vi "Siglent SDG X Series Frequency Sweep.vi"() -> ()   [LabVIEW 2022 SP3]
doc: "This example shows how to configure and enable a frequency sweep."
uses:
  Siglent SDG X Series.lvlib
panel:
  in  "VISA resource name":refnum<visa-resource-name>
  in  "Stop Frequency  (1000.0 Hz)":dbl=1000.0 format="%#.6g"
  in  "Start Frequency (100.0 Hz)":dbl=100.0 format="%#.6g"
  in  "Sweep Time (1.00 s)":dbl=1.0 format="%#.6g"
  in  "Amplitude (1.0 Vpp)":dbl=1.0 format="%#.3f"
  in  "Waveform Function (0: Sine)":u16(ring) items=["Sine", "Square", "Ramp", "DC", "Pulse", "Arb"]
  in  "Channel (1:Channel 1)":i32(ring)=1 items=["Channel 1"=1, "Channel 2"=2]
  # "(c) 2017 SIGLENT TECHNOLOGIES CO.,LTD. ALL RIGHTS RESERVED."
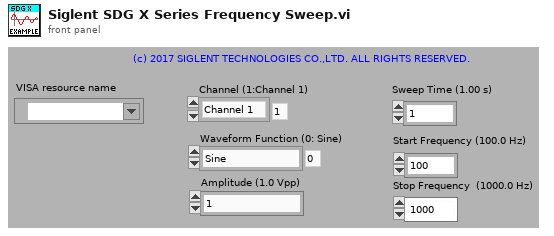
[diagram p1: front panel]
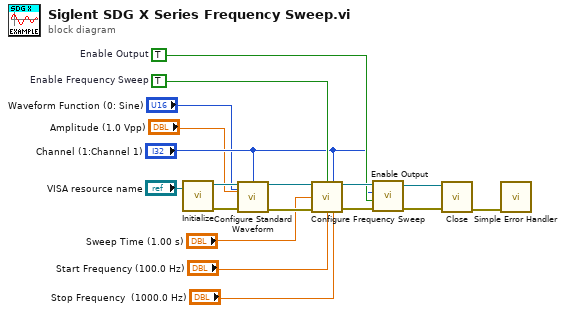
[diagram p0: block diagram]
diagram:
  w8 = TRUE  # Enable Output
  w13 = TRUE  # Enable Frequency Sweep
  n1 = call "Initialize.vi"("VISA resource name"="VISA resource name") -> ("error out"=w14:errorcluster, "VISA resource name out"=w18:refnum<visa-resource-name>)  [unwired: 9 in]
  n2 = call "Configure Standard Waveform.vi"("VISA resource name"=w18, "Waveform Function (0: Sine)"="Waveform Function (0: Sine)", "Channel (1:Channel 1)"="Channel (1:Channel 1)", "Amplitude (1.0 Vpp)"="Amplitude (1.0 Vpp)", "error in (no error)"=w14) -> ("VISA resource name out"=w15:refnum<visa-resource-name>, "error out"=w16:errorcluster)  [unwired: 9 in]
  n3 = call "Configure Frequency Sweep.vi"("VISA resource name"=w15, "Enable Frequency Sweep (T:Enable)"=w13, "Channel (1:Channel 1)"="Channel (1:Channel 1)", "Sweep Time (1.00 s)"="Sweep Time (1.00 s)", "error in (no error)"=w16, "Start Frequency (100.0 Hz)"="Start Frequency (100.0 Hz)", "Stop Frequency  (1000.0 Hz)"="Stop Frequency  (1000.0 Hz)") -> ("VISA resource name out"=w12:refnum<visa-resource-name>, "error out"=w11:errorcluster)  [unwired: 7 in]
  n4 = call "Enable Output.vi"("error in (no error)"=w11, "Enable Output (T: Enable)"=w8, "Channel (1:Channel 1)"="Channel (1:Channel 1)", "VISA resource name"=w12) -> ("error out"=w10:errorcluster, "VISA resource name out"=w9:refnum<visa-resource-name>)  [unwired: 6 in]
  n5 = call "Close.vi"("error in (no error)"=w10, "VISA resource name"=w9) -> ("error out"=w17:errorcluster)  [unwired: 9 in]
  n6 = call <vilib>:"Simple Error Handler.vi"("error in (no error)"=w17) -> ()  [unwired: 4 in, 5 out]
